vi "Validate Response Refnum.vi"(8 "error in (no error)":errorcluster, 11 "response refnum in":T1 format="%.0x") -> (0 "error out":errorcluster, 3 "response refnum out":u64)   [LabVIEW 2018, in "Instrument Addon Scripting API.lvlib"]
uses:
  Instrument Addon Scripting API.lvlib
  <vilib>/NI Veristand/Custom Device API/Custom Device Item Ref.ctl
  Addon/Addon Shared/SubVIs/Constants.vi
  <vilib>/Utility/error.llb/Error Cluster From Error Code.vi
  <vilib>/ErrorRing/Error Ring.xnode
  <vilib>/NI/NI VeriStand Advanced SysDef API/SysDef API/Advanced System Definition.lvlib
  Addon/Addon Shared/Instrument Addon Shared.lvlib
  <vilib>/NI Veristand/Custom Device API/Custom Device API.lvlib
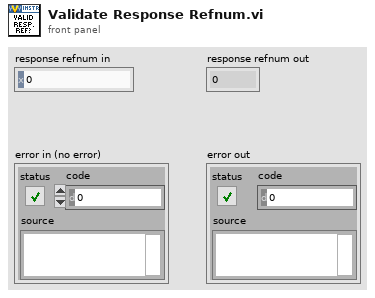
[diagram p1: front panel]
types:
  T1 = typedef "Custom Device API.lvlib/Custom Device Item Ref.ctl" = u64
  T2 = typedef "Advanced System Definition.lvlib/TreeItem.Info.ctl" = cluster{"Name":string, "Description":string, "GUID":string, "Is Channel":bool, "Channel":T3, "Is Waveform":bool, "Waveform":T5}
  T3 = typedef "Custom Device API.lvlib/Custom Device Channel.ctl" = cluster{"Type":T4, "Units":string, "Default Value":dbl, "Faultable":bool, "Scalable":bool}
  T4 = typedef "Custom Device API.lvlib/Custom Device Channel Type.ctl" = enum16{"Input", "Output"}
  T5 = typedef "Custom Device API.lvlib/Custom Device Waveform.ctl" = cluster{"Data Type":T6, "Units":string}
  T6 = typedef "Custom Device API.lvlib/Custom Device Waveform DataType.ctl" = enum16{"Double", "Complex Double"}
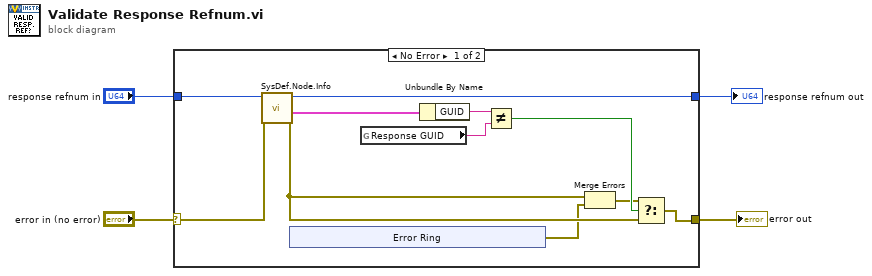
[diagram p0: block diagram]
diagram:
  n1 = case shown="No Error" "error in (no error)" {
    selector: "error in (no error)" -> [w9 w21]
    tunnel: [w13 w22] -> w4
    tunnel: "response refnum in" -> [w11 w22]
    tunnel: [w8 w21] -> w1
    frame No Error {
      n2 = call <vilib>:"SysDef.Node.Info.vi"("error in (no error)"=w9, "nodeID"=w11) -> ("error out"=w6:errorcluster, "Item Info"=w12:T2, "nodeID out"=w13:u64)  [unwired: 6 in, 1 out]
      n3 = xnode "Error Ring"() -> ("error out"=w5:errorcluster)
      n4 = global read "Constants.vi" "Response GUID"() -> (w15:string)
      n5 = Unbundle By Name(w12) -> ("GUID"=w14:string)
      n6 = Not Equal?(x=w14, y=w15) -> (x != y?=w10:bool)
      n7 = Merge Errors(w6, w5) -> (w7:errorcluster)
      n8 = Select(t=w7, s=w10, f=w6) -> (s? t:f=w8:errorcluster)
    }
    frame Error {
    }
  }
  "response refnum out" <- w4
  "error out" <- w1
